vi "Create_Arbirary_Signal.vi"() -> ()   [LabVIEW 2022 SP3]
uses:
  <vilib>/Analysis/1siggen.llb/Ramp Pattern by Samples.vi
  <vilib>/Analysis/NI_AALPro.lvlib
  <vilib>/Analysis/NI_AALBase.lvlib
panel:
  out "Ramp Pattern":dbl[](array[numeric])
  out "XY Graph":cluster{"X":dbl[], "Ramp Pattern":dbl[]}(graph)
  in  "Amp Spectrum Phase (radians)":dbl[](array[numeric])
  in  "Amp Spectrum Mag (Vrms)":dbl[](array[numeric])
  in  "Freq":dbl=620.69
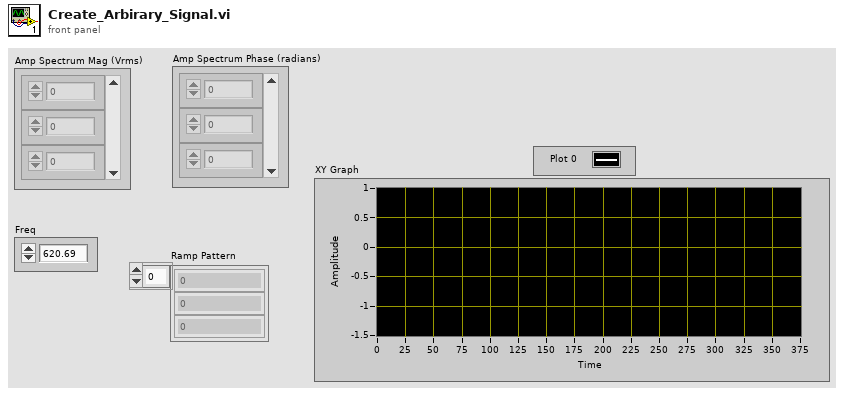
[diagram p1: front panel]
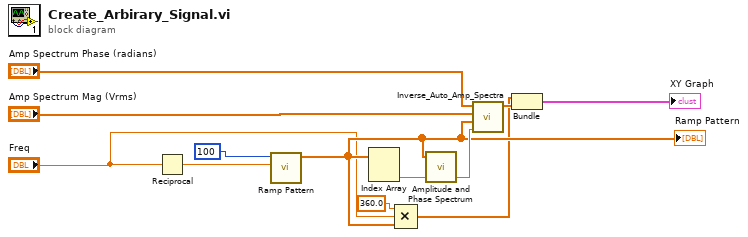
[diagram p0: block diagram]
diagram:
  n1 = Reciprocal(x="Freq") -> (1/x=w7:dbl)
  n2 = call-poly <vilib>:"Ramp Pattern.vi"("end"=w7, "samples"=100) -> ("Ramp Pattern"=w4:dbl[])  [unwired: 8 in, 1 out]
  "Ramp Pattern" <- w4
  n3 = Index Array(array=w4) -> (element #2=w11:dbl)  [unwired: 2 in, 1 out]
  n4 = Compound Arithmetic op=MULTIPLY(360.0 ("value"), "Freq", w4) -> (w1:dbl[])
  n5 = call <vilib>:"Amplitude and Phase Spectrum.vi"("dt"=w11, "Signal (V)"=w4) -> ("df"=w5:dbl)  [unwired: 1 in, 2 out]
  n6 = call "Inverse_Auto_Amp_Spectra.vi"("df"=w5, "t"=w4, "Amp Spectrum Mag (Vrms)"="Amp Spectrum Mag (Vrms)", "Amp Spectrum Phase (radians)"="Amp Spectrum Phase (radians)") -> ("X"=w6:dbl[])  [unwired: 6 in, 1 out]
  n7 = Bundle(w1, "X"=w6) -> (→"XY Graph":cluster{dbl[], "X":dbl[]})  [unwired: 1 in]
